vi "DeltaE(1994).vi"(1 "L*a*b colors":T1, 2 "Surface Type":bool) -> (0 "Delta E":dbl)   [LabVIEW 2013]
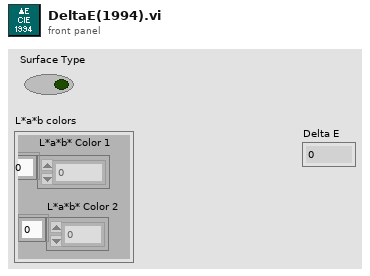
[diagram p1: front panel]
types:
  T1 = cluster{"L*a*b* Color 1":dbl[], "L*a*b* Color 2":dbl[]}
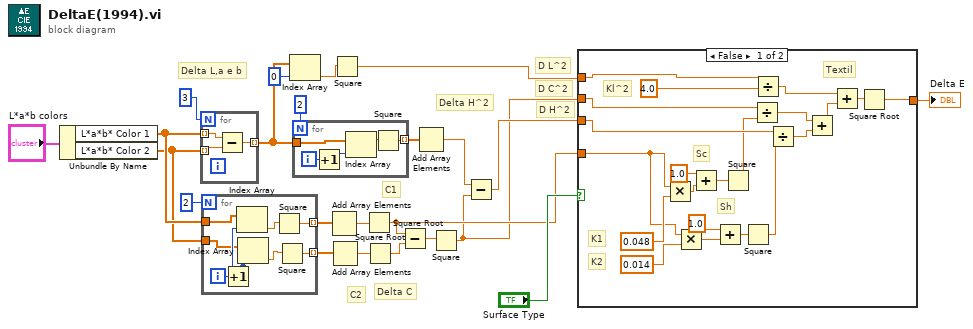
[diagram p0: block diagram]
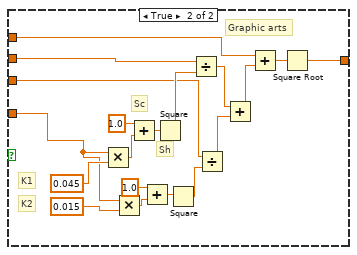
[diagram p2: hidden frame]
diagram:
  # "D H^2"
  # "D C^2"
  # "D L^2"
  # "Delta H^2"
  # "Delta C"
  # "C2"
  # "C1"
  # "Delta L,a e b"
  n1 = Unbundle By Name("L*a*b colors") -> ("L*a*b* Color 1"=w20:dbl[], "L*a*b* Color 2"=w19:dbl[])
  n2 = for {
    N: 3 -> [_]
    tunnel: w20 -> [w26] mode=indexing
    tunnel: w19 -> [w25] mode=indexing
    tunnel: [w24] -> w5 mode=indexing
    n3 = Subtract(x=w26, y=w25) -> (x-y=w24:dbl)
  }
  n4 = for {
    N: 2 -> [_]
    tunnel: w20 -> [w33]
    tunnel: w19 -> [w31]
    tunnel: [w28] -> w18 mode=indexing
    tunnel: [w27] -> w17 mode=indexing
    i -> [w34]
    n5 = Increment(x=w34) -> (x+1=w32:i32)
    n6 = Index Array(array=w33, index=w32) -> (element=w30:dbl)
    n7 = Index Array(array=w31, index=w32) -> (element=w29:dbl)
    n8 = Square(x=w30) -> (x^2=w28:dbl)
    n9 = Square(x=w29) -> (x^2=w27:dbl)
  }
  n10 = Index Array(array=w5, index=0) -> (element=w3:dbl)
  n11 = for {
    N: 2 -> [_]
    tunnel: w5 -> [w38]
    tunnel: [w35] -> w12 mode=indexing
    i -> [w39]
    n12 = Increment(x=w39) -> (x+1=w37:i32)
    n13 = Index Array(array=w38, index=w37) -> (element=w36:dbl)
    n14 = Square(x=w36) -> (x^2=w35:dbl)
  }
  n15 = Add Array Elements(numeric array=w18) -> (sum=w16:dbl)
  n16 = Add Array Elements(numeric array=w17) -> (sum=w15:dbl)
  n17 = Square(x=w3) -> (x^2=w2:dbl)
  n18 = Square Root(x=w16) -> (sqrt(x)=w8:dbl)
  n19 = Square Root(x=w15) -> (sqrt(x)=w14:dbl)
  n20 = Subtract(x=w8, y=w14) -> (x-y=w11:dbl)
  n21 = Add Array Elements(numeric array=w12) -> (sum=w10:dbl)
  n22 = Square(x=w11) -> (x^2=w6:dbl)
  n23 = Subtract(x=w10, y=w6) -> (x-y=w7:dbl)
  n24 = case shown="False" "Surface Type" {
    tunnel: w8 -> [w55 w75]
    tunnel: w7 -> [w51 w67]
    tunnel: w6 -> [w49 w70]
    tunnel: w2 -> [w47 w63]
    tunnel: [w40 w61] -> w1
    frame False {
      # "Sh"
      # "Sc"
      # "K1"
      # "K2"
      # "Kl^2"
      # "Textil"
      n25 = Multiply(x=w55, y=0.048) -> (x*y=w59:dbl)
      n26 = Multiply(x=w55, y=0.014) -> (x*y=w57:dbl)
      n27 = Add(x=1.0, y=w59) -> (x+y=w53:dbl)
      n28 = Add(x=1.0, y=w57) -> (x+y=w52:dbl)
      n29 = Square(x=w53) -> (x^2=w48:dbl)
      n30 = Square(x=w52) -> (x^2=w50:dbl)
      n31 = Divide(x=w49, y=w48) -> (x/y=w44:dbl)
      n32 = Divide(x=w47, y=4.0) -> (x/y=w43:dbl)
      n33 = Divide(x=w51, y=w50) -> (x/y=w45:dbl)
      n34 = Add(x=w44, y=w45) -> (x+y=w42:dbl)
      n35 = Add(x=w43, y=w42) -> (x+y=w41:dbl)
      n36 = Square Root(x=w41) -> (sqrt(x)=w40:dbl)
    }
    frame True {
      # "Sh"
      # "Sc"
      # "K1"
      # "K2"
      # "Graphic arts"
      n37 = Multiply(x=w75, y=0.045) -> (x*y=w77:dbl)
      n38 = Multiply(x=w75, y=0.015) -> (x*y=w73:dbl)
      n39 = Add(x=1.0, y=w77) -> (x+y=w71:dbl)
      n40 = Add(x=1.0, y=w73) -> (x+y=w72:dbl)
      n41 = Square(x=w71) -> (x^2=w69:dbl)
      n42 = Square(x=w72) -> (x^2=w68:dbl)
      n43 = Divide(x=w70, y=w69) -> (x/y=w66:dbl)
      n44 = Divide(x=w67, y=w68) -> (x/y=w65:dbl)
      n45 = Add(x=w66, y=w65) -> (x+y=w64:dbl)
      n46 = Add(x=w63, y=w64) -> (x+y=w62:dbl)
      n47 = Square Root(x=w62) -> (sqrt(x)=w61:dbl)
    }
  }
  "Delta E" <- w1
